vi "AnalogIntegratorFastOszi_NI5751.vi"() -> ()   [LabVIEW 2012]
uses:
  <vilib>/eio/EIONode/EIONode.xnode
  <vilib>/rvi/eio/common/nirviEmuTemplateMethod_errors.vi
  <vilib>/Platform/TimedLoop/XDataNode/wakeup.ctl
  <vilib>/Platform/TimedLoop/XDataNode/XDNodeRunTimeDep.lvlib
  <vilib>/Platform/TimedLoop/XDataNode/nitl_modes.ctl
  <vilib>/Platform/TimedLoop/XDataNode/timing_clust.ctl
  <vilib>/Platform/TimedLoop/XDataNode/XDataNode.xnode
  <vilib>/rvi/DataTransferAndStorage/Container/XNode/niFpgaContainer.xnode
  <vilib>/rvi/FIFO/Fifo_Resource/nirvififoEmulationWrite.vi
  <vilib>/rvi/FIFO/Fifo_Resource/nirvififoEmulationClear.vi
  <vilib>/rvi/FIFO/Fifo_Resource/nirvififoEmulationRead.vi
  <vilib>/rvi/interface/RandomDataEmulation/nirviRandomDataFpgaReadWriteTemplate.vi
panel:
  in  "Acquire continuously":bool
  in  "Clear Interloop FIFO":bool
  out "InterloopFIFO Timeout":bool
  out "ToHostCh1FIFO Overflow":bool
  in  "Acquire":bool
  out "InterloopFIFO Overflow":bool
  out "Acquiring":bool
  out "IO Module\\AI Over Range":bool
  in  "Samples to acquire":u32=10000 caption="Samples per pixel Acq"
  out "Configured?":bool
  # "5771 IO module configuration"
  # "Analog integrator Fast Oszi mode"
  # "Acquisition control"
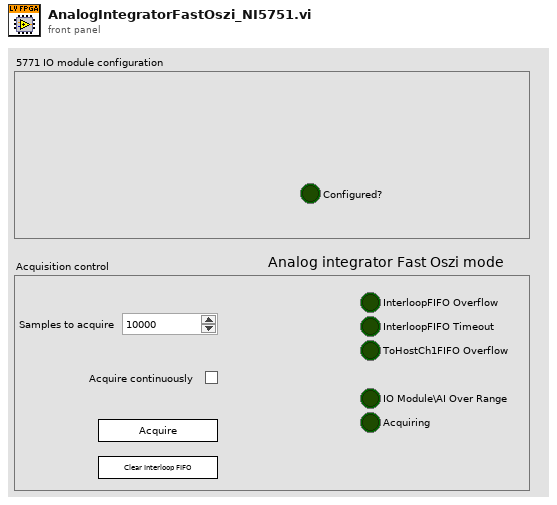
[diagram p1: front panel]
types:
  T1 = typedef "XDNodeRunTimeDep.lvlib/timing_clust.ctl" = cluster{"Expected End [f-1]":u64, "Actual End [f-1]":u64, "Finished Late? [f-1]":bool, "Expected End [i-1]":u64, "Actual End [i-1]":u64, "Finished Late? [i-1]":bool, "Expected Start [i]":u64, "Actual Start [i]":u64, "Expected Start [f]":u64, "Actual Start [f]":u64, "Source Name":string, "Structure Name":string, "Period":i64, "Deadline":i64, "Offset":i64, "Start":i64, "Priority":i32, "Timeout":i32, "Mode":T2, "Wakeup Reason":T3, "Error":errorcluster, "Source Type":string, "Secondary Source Type":string, "Global End Time":u64, "Global Start Time":u64, "Frame Duration":u64, "Iteration Duration":u64, "Assigned CPU":i32, "I/O Scan Engine Mode":u32}
  T2 = typedef "XDNodeRunTimeDep.lvlib/nitl_modes.ctl" = enum32{"No Change", "Process missed periods, maintain original phase", "Discard missed periods, maintain original phase", "Process missed periods, ignore original phase", "Discard missed periods, ignore original phase"}
  T3 = typedef "XDNodeRunTimeDep.lvlib/wakeup.ctl" = enum32{"Normal", "Aborted", "Asynchronous wakeup", "Timing source error", "Timed loop error", "Timeout"}
  T4 = cluster{u64, "IO Module\\Synchronous Trigger Input":void}
  T5 = cluster{"Data U64":u64, "IO Module\\Synchronous Trigger Input":u8}
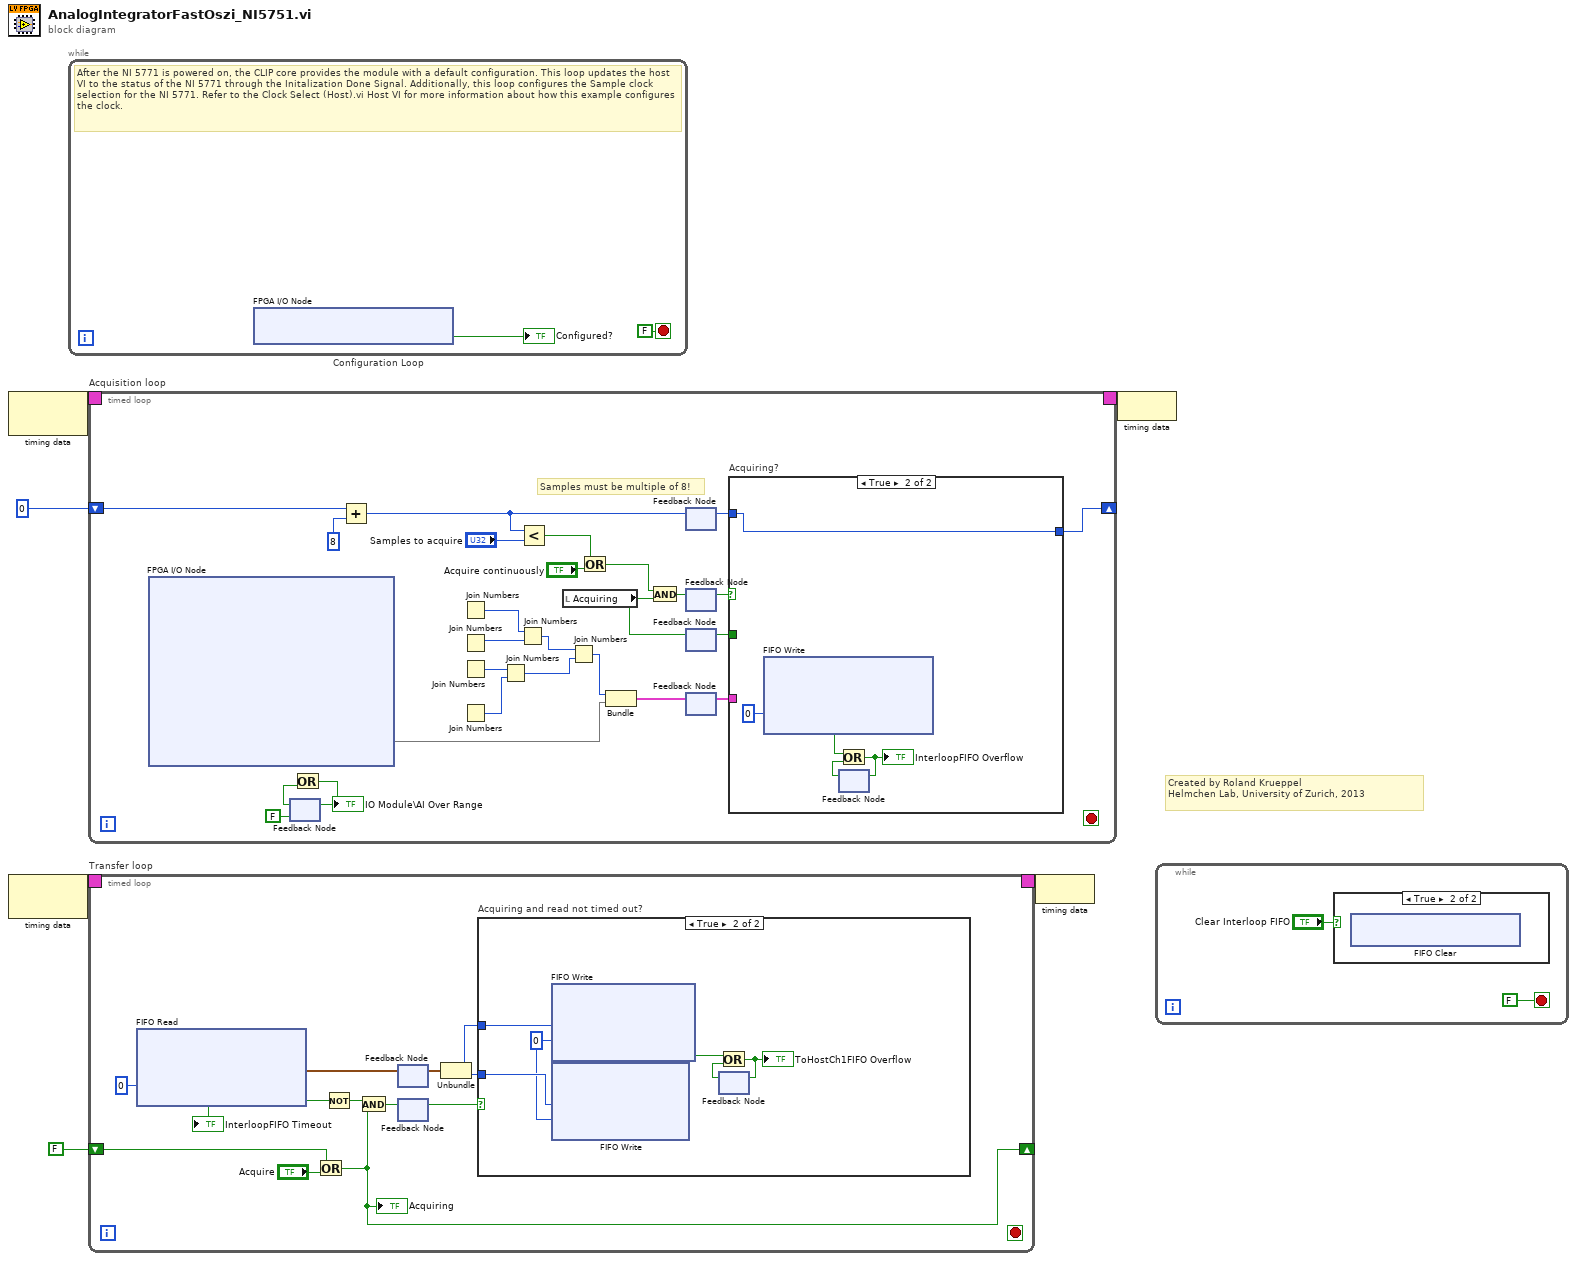
[diagram p0: block diagram]
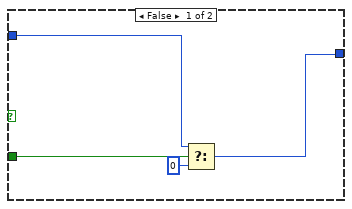
[diagram p4: hidden frame]
diagram:
  # "Created by Roland Krueppel\nHelmchen Lab, University of Zurich, 2013"
  n1 = node-c288() -> (w6:T1)  [unwired: 1 in]
  n2 = node-c288() -> (w3:T1)  [unwired: 1 in]
  n3 = while "Configuration Loop" {
    stop <- FALSE stop-if-true
    # "After the NI 5771 is powered on, the CLIP core provides the module with a default configuration. This loop updates the host VI to the status of the NI 5771 through the Initalization Done Signal. Additionally, this loop configures the Sample clock selection for the NI 5771. Refer to the Clock Select (Host).vi Host VI for more information about how this example configures the clock."
    n4 = xnode "FPGA I/O Node"() -> ("IO Module\\Initialization Done"=→"Configured?":bool)  [unwired: 1 in, 1 out]
  }
  n5 = timed-loop "Acquisition loop" {
    timing: w6 -> [_]
    timing-out: [_] -> w5
    shift-right: [w31] -> _
    shift-left: u32 0 ("t") -> [w28]
    stop <- _ stop-if-true
    # "Samples must be multiple of 8!"
    n6 = xnode "FPGA I/O Node"() -> ("IO Module\\Synchronous Trigger Input"=w20)  [unwired: 10 in, 19 out]
    n7 = feedback #1(FALSE) -> (w34:bool)
    n8 = Or(y=w34) -> (x .or. y?=w33:bool)  [unwired: 1 in]
    "IO Module\\AI Over Range" <- w33
    n9 = feedback-in #1(w33) -> ()
    n10 = Add(x=w28, y=u32 8) -> (x+y=w17:u32)
    n11 = Join Numbers() -> ((hi.lo)=w27:u32)  [unwired: 2 in]
    n12 = Join Numbers() -> ((hi.lo)=w26:u32)  [unwired: 2 in]
    n13 = Join Numbers() -> ((hi.lo)=w25:u32)  [unwired: 2 in]
    n14 = Join Numbers() -> ((hi.lo)=w24:u32)  [unwired: 2 in]
    n15 = Join Numbers(hi=w25, lo=w24) -> ((hi.lo)=w22:u64)
    n16 = Join Numbers(hi=w27, lo=w26) -> ((hi.lo)=w23:u64)
    n17 = Less?(x=w17, y="Samples to acquire") -> (x < y?=w11:bool)
    n18 = local read "Acquiring"() -> (w13:bool)
    n19 = Join Numbers(hi=w23, lo=w22) -> ((hi.lo)=w21:u64)
    n20 = Or(x=w11, y="Acquire continuously") -> (x .or. y?=w9:bool)
    n21 = Bundle(w21, "IO Module\\Synchronous Trigger Input"=w20) -> (w19:T4)  [unwired: 1 in]
    n22 = And(x=w9, y=w13) -> (x .and. y?=w15:bool)
    n23 = feedback #2() -> (w16:u32)  [unwired: 1 in]
    n24 = feedback-in #2(w17) -> ()
    n25 = feedback #3() -> (w14:bool)  [unwired: 1 in]
    n26 = feedback-in #3(w15) -> ()
    n27 = feedback #4() -> (w12:bool)  [unwired: 1 in]
    n28 = feedback-in #4(w13) -> ()
    n29 = feedback #5() -> (w18:T4)  [unwired: 1 in]
    n30 = feedback-in #5(w19) -> ()
    n31 = case "Acquiring?" shown="True" w14 {
      tunnel: [w35 w39] -> w31
      tunnel: w18 -> [_ _]
      tunnel: w16 -> [w37 w39]
      tunnel: w12 -> [w38 _]
      frame False {
        n32 = Select(t=w37, s=w38, f=u16 0 ("t")) -> (s? t:f=w35:u32)
      }
      frame True {
        n33 = xnode ("FIFO Write")("Timeout"=0) -> ("Timed Out?"=w42:bool)  [unwired: 2 in, 1 out]
        n34 = feedback #6() -> (w40:bool)  [unwired: 1 in]
        n35 = Or(x=w42, y=w40) -> (x .or. y?=w41:bool)
        "InterloopFIFO Overflow" <- w41
        n36 = feedback-in #6(w41) -> ()
      }
    }
  }
  n37 = timed-loop "Transfer loop" {
    timing: w3 -> [_]
    timing-out: [_] -> w2
    shift-right: [w54] -> _
    shift-left: FALSE -> [w52]
    stop <- _ stop-if-true
    n38 = xnode ("FIFO Read")("Timeout"=0) -> ("Element"=w49:T5, "Timed Out?"=w56:bool)  [unwired: 1 in, 1 out]
    "InterloopFIFO Timeout" <- w56
    n39 = Or(x=w52, y="Acquire") -> (x .or. y?=w54:bool)
    "Acquiring" <- w54
    n40 = Not(x=w56) -> (.not. x?=w55:bool)
    n41 = And(x=w55, y=w54) -> (x .and. y?=w47:bool)
    n42 = feedback-in #7(w49) -> ()
    n43 = feedback #7() -> (w48:T5)  [unwired: 1 in]
    n44 = feedback #8() -> (w46:bool)  [unwired: 1 in]
    n45 = feedback-in #8(w47) -> ()
    n46 = Unbundle(w48) -> ("Data U64"=w51:u64, "IO Module\\Synchronous Trigger Input"=w50:u8)
    n47 = case "Acquiring and read not timed out?" shown="True" w46 {
      tunnel: w51 -> [_ w60]
      tunnel: w50 -> [_ w59]
      frame False {
      }
      frame True {
        w58 = 0 ("Timeout")
        n48 = xnode ("FIFO Write")("Element"=w60, "Timeout"=w58) -> ("Timed Out?"=w62:bool)  [unwired: 1 in, 1 out]
        n49 = xnode ("FIFO Write")("Element"=w59, "Timeout"=w58) -> ()  [unwired: 1 in, 2 out]
        n50 = feedback #9() -> (w61:bool)  [unwired: 1 in]
        n51 = Or(x=w62, y=w61) -> (x .or. y?=w63:bool)
        "ToHostCh1FIFO Overflow" <- w63
        n52 = feedback-in #9(w63) -> ()
      }
    }
  }
  n53 = node-c288(w2) -> ()
  n54 = node-c288(w5) -> ()
  n55 = while {
    stop <- FALSE stop-if-true
    n56 = case shown="True" "Clear Interloop FIFO" {
      frame False {
      }
      frame True {
        n57 = xnode ("FIFO Clear")() -> ()  [unwired: 1 in, 1 out]
      }
    }
  }
